vi "mirrorCorrections.vi"(0 "Scan Mirror Min":T3 min=-10.0 max=10.0, 1 "Beam@maxZ":T3 min=-10.0 max=10.0, 2 "Z Mirror Offset":T2, 3 "Z Mirror Gain":T1, 4 "Piezo Position (µm)":T4 min=0.0 max=100.0, 5 "Piezo Min (µm)":T4 min=0.0 max=100.0, 6 "Piezo Max (µm)":T4 min=0.0 max=100.0, 8 "Scan Mirror Max":T3 min=-10.0 max=10.0, 10 "Scan Mirror Voltage":T3 min=-10.0 max=10.0, 11 "Scan Mirror Position 2":T3 min=-10.0 max=10.0, 12 "Z Mirror Control":enum16{"manual", "automatic"}(ring), 13 "Z Offset Position 2":T2, 14 "Apply ex/det correction":enum16{"no", "yes"}(ring)) -> (21 "Adjusted Scan Mirror Voltage":T3 min=-10.0 max=10.0, 25 "Z Mirror Voltage":T3 min=-10.0 max=10.0)   [LabVIEW 2013]
uses:
  Mirror_Voltage.ctl
  Piezo_micrometres.ctl
  Z_Offset.ctl
  Gain.ctl
panel:
  out "localCalibrationGain":dbl
  out "deltaZ":dbl
  out "scanMirrorCentrePosition":dbl
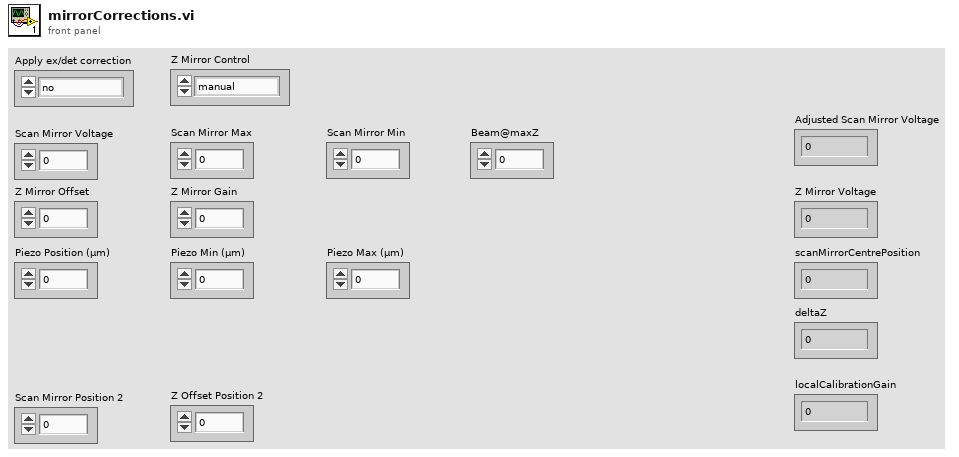
[diagram p1: front panel]
types:
  T1 = typedef "Gain.ctl" = dbl
  T2 = typedef "Z_Offset.ctl" = dbl
  T3 = typedef "Mirror_Voltage.ctl" = dbl
  T4 = typedef "Piezo_micrometres.ctl" = dbl
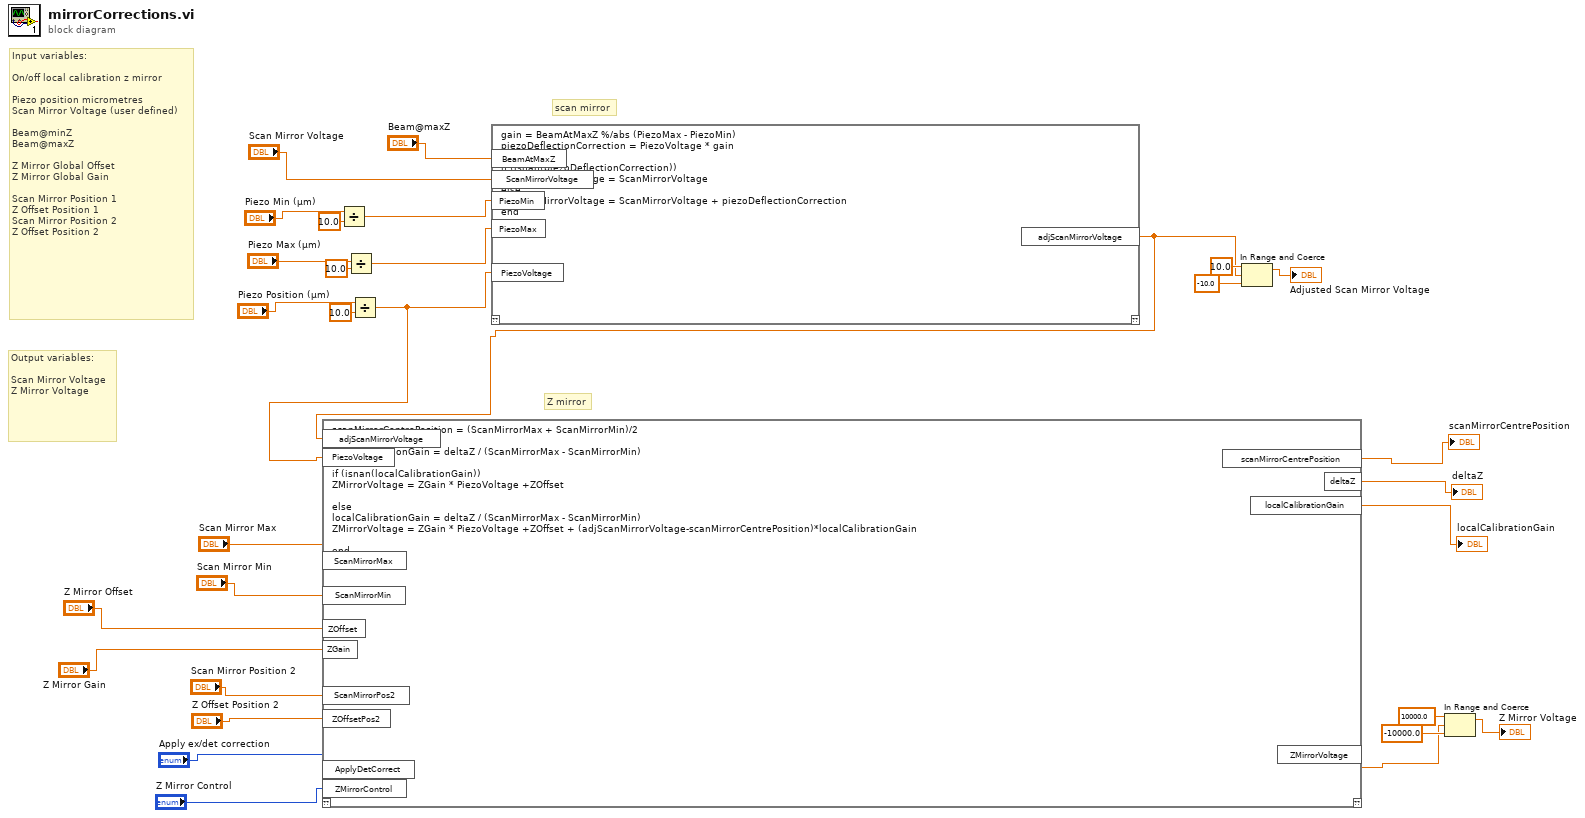
[diagram p0: block diagram]
diagram:
  # "Z mirror"
  # "scan mirror"
  # "Output variables:\n\nScan Mirror Voltage\nZ Mirror Voltage"
  # "Input variables:\n\nOn/off local calibration z mirror\n\nPiezo position micrometres\nScan Mirror Voltage (user defined)\n\nBeam@minZ\nBeam@maxZ\n\nZ Mirror Global Offset\nZ Mirror Global Gain\n\nScan Mirror Position 1\nZ Offset Position 1\nScan Mirror Position 2\nZ Offset Position 2"
  n1 = Divide(x="Piezo Min (µm)", y=10.0) -> (x/y=w22:T4)
  n2 = Divide(x="Piezo Max (µm)", y=10.0) -> (x/y=w21:T4)
  n3 = Divide(x="Piezo Position (µm)", y=10.0) -> (x/y=w15:T4)
  n4 = mathscript code="gain = BeamAtMaxZ %/abs (PiezoMax - PiezoMin)\npiezoDeflectionCorrection = PiezoVoltage * gain\n\nif (isnan(piezoDeflectionCorrection))\nadjScanMirrorVoltage = ScanMirrorVoltage \nelse\nadjScanMirrorVoltage = ScanMirrorVoltage + piezoDeflectionCorrection\nend"("BeamAtMaxZ"="Beam@maxZ", "ScanMirrorVoltage"="Scan Mirror Voltage", "PiezoMin"=w22, "PiezoMax"=w21, "PiezoVoltage"=w15) -> ("adjScanMirrorVoltage"=w8:dbl)  [unwired: 1 in, 1 out]
  n5 = mathscript code="scanMirrorCentrePosition = (ScanMirrorMax + ScanMirrorMin)/2\ndeltaZ  = ZOffsetPos2 \nlocalCalibrationGain = deltaZ / (ScanMirrorMax - ScanMirrorMin)\n\nif (isnan(localCalibrationGain))\nZMirrorVoltage = ZGain * PiezoVoltage +ZOffset\n\nelse\nlocalCalibrationGain = deltaZ / (ScanMirrorMax - ScanMirrorMin)\nZMirrorVoltage = ZGain * PiezoVoltage +ZOffset + (adjScanMirrorVoltage-scanMirrorCentrePosition)*localCalibrationGain\n\nend"("PiezoVoltage"=w15, "adjScanMirrorVoltage"=w8, "ScanMirrorMax"="Scan Mirror Max", "ScanMirrorMin"="Scan Mirror Min", "ScanMirrorPos2"="Scan Mirror Position 2", "ZOffsetPos2"="Z Offset Position 2", "ApplyDetCorrect"="Apply ex/det correction", "ZMirrorControl"="Z Mirror Control", "ZOffset"="Z Mirror Offset", "ZGain"="Z Mirror Gain") -> ("ZMirrorVoltage"=w5:dbl, "scanMirrorCentrePosition"=→"scanMirrorCentrePosition":dbl, "deltaZ"=→"deltaZ":dbl, "localCalibrationGain"=→"localCalibrationGain":dbl)  [unwired: 1 in, 1 out]
  n6 = In Range and Coerce(upper limit=10.0, x=w8, lower limit=-10.0) -> (coerced(x)=→"Adjusted Scan Mirror Voltage":dbl)  [unwired: 1 out]
  n7 = In Range and Coerce(upper limit=10000.0, x=w5, lower limit=-10000.0) -> (coerced(x)=→"Z Mirror Voltage":dbl)  [unwired: 1 out]
